vi "SVP Saturated Vapor pressure (Pa).vi"(1 "Tceg":dbl[unit]) -> (0 "SVP":dbl[unit])   [LabVIEW 2018]
panel:
  out "SVP\nVapor Pressure(Pa)\nSVP=(10**5)*(EXP**(11.78*(Tk-372.79)/(Tk-43.15)));":dbl[unit](knob)
  out "Temprature Of Input Air\nKelvin Degree":dbl[unit](slide) scale=273.0..373.0
  out "Tk":dbl[unit]
  out "Temprature Of Input Air\nCentigrade Degree":dbl[unit](slide) scale=0.0..100.0
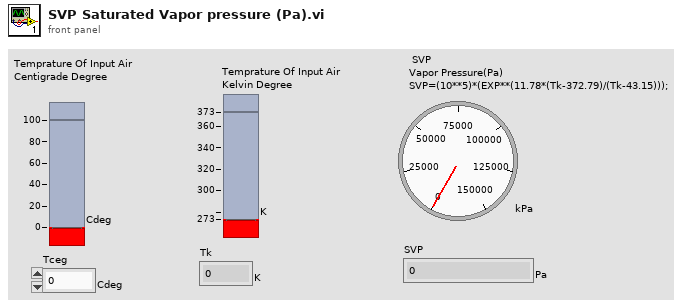
[diagram p1: front panel]
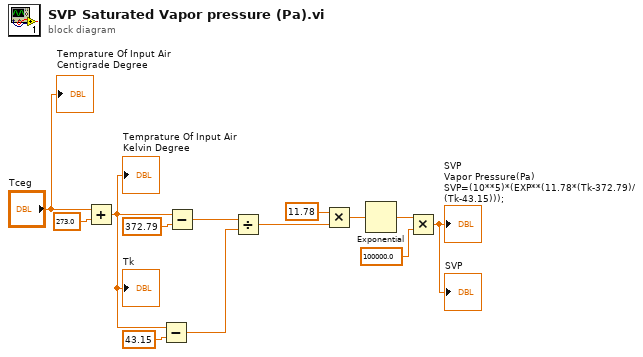
[diagram p0: block diagram]
diagram:
  n1 = Add(x="Tceg", y=dbl[unit] 273.0) -> (x+y=w1:dbl[unit])
  "Tk" <- w1
  "Temprature Of Input Air\nKelvin Degree" <- w1
  n2 = Subtract(x=w1, y=dbl[unit] 43.15) -> (x-y=w3:dbl[unit])
  n3 = Subtract(x=w1, y=dbl[unit] 372.79) -> (x-y=w6:dbl[unit])
  n4 = Divide(x=w6, y=w3) -> (x/y=w8:dbl)
  n5 = Multiply(x=11.78, y=w8) -> (x*y=w7:dbl)
  n6 = Exponential(1:w7) -> (0:w10:dbl)
  n7 = Multiply(x=w10, y=dbl[unit] 100000.0) -> (x*y=→"SVP\nVapor Pressure(Pa)\nSVP=(10**5)*(EXP**(11.78*(Tk-372.79)/(Tk-43.15)));" →"SVP":dbl[unit])
  "Temprature Of Input Air\nCentigrade Degree" <- "Tceg"
